vi "Get Available IP List.vi"(7 "ip list property name":string, 8 "error in (no error)":errorcluster, 11 "Item Ref in":T1 format="%.0x") -> (0 "error out":errorcluster, 2 "ips available":string[](array[string]), 3 "Item Ref out":T1 format="%.0x")   [LabVIEW 2017, in "Engine Simulation Toolkit System Explorer.lvlib"]
uses:
  Engine Simulation Toolkit System Explorer.lvlib
  <vilib>/NI Veristand/Custom Device API/Custom Device Item Ref.ctl
  <vilib>/NI Veristand/Custom Device Tools/Custom Device Utility Library/Search Direction.ctl
  Shared/Constants and GUIDs.vi
  <vilib>/NI Veristand/Custom Device Tools/Custom Device Utility Library/NI VeriStand - Search for Item by GUID.vi
  <vilib>/NI Veristand/Custom Device API/Get Item Property (String Array).vi
  <vilib>/NI Veristand/Custom Device Tools/Custom Device Utility Library/Custom Device Utility Library.lvlib
  Shared/Engine Simulation Toolkit Shared.lvlib
  <vilib>/NI Veristand/Custom Device API/Custom Device API.lvlib
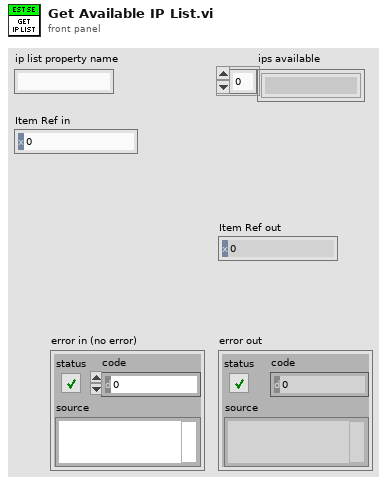
[diagram p1: front panel]
types:
  T1 = typedef "Custom Device API.lvlib/Custom Device Item Ref.ctl" = u64
  T2 = typedef "Custom Device Utility Library.lvlib/Search Direction.ctl" = enum16{"Down", "Up"}
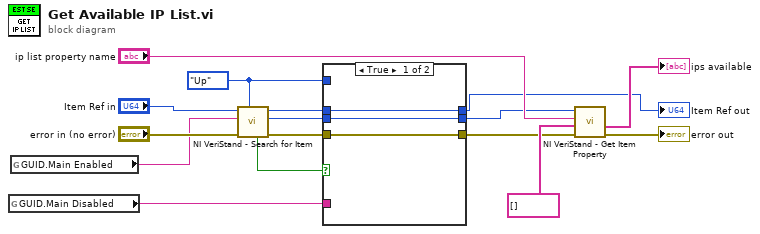
[diagram p0: block diagram]
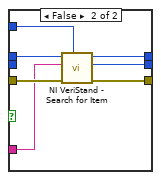
[diagram p2: hidden frame]
diagram:
  w4 = Search_Direction."Up" ("Direction (Down)")
  n1 = global read "Constants and GUIDs.vi" "GUID.Main Disabled"() -> (w5:string)
  n2 = global read "Constants and GUIDs.vi" "GUID.Main Enabled"() -> (w14:string)
  n3 = call-poly <vilib>:"NI VeriStand - Search for Item.vi"("Direction (Down)"=w4, "error in"="error in (no error)", "Item GUID"=w14, "Section Ref in"="Item Ref in") -> ("error out"=w8:errorcluster, "Item Ref"=w6:T1, "Section Ref out"=w7:T1, "Found"=w9:bool)  [unwired: 4 in]
  n4 = case shown="True" w9 {
    tunnel: w8 -> [w19 w26]
    tunnel: w7 -> [w17 w25]
    tunnel: w6 -> [w18 _]
    tunnel: w5 -> [_ w24]
    tunnel: w4 -> [_ w23]
    tunnel: [w18 w22] -> w3
    tunnel: [w17 w21] -> w2
    tunnel: [w19 w20] -> w1
    frame True {
    }
    frame False {
      n5 = call-poly <vilib>:"NI VeriStand - Search for Item.vi"("Direction (Down)"=w23, "error in"=w26, "Item GUID"=w24, "Section Ref in"=w25) -> ("error out"=w20:errorcluster, "Item Ref"=w22:T1, "Section Ref out"=w21:T1)  [unwired: 4 in, 1 out]
    }
  }
  "Item Ref out" <- w2
  n6 = call-poly <vilib>:"NI VeriStand - Get Item Property.vi"("error in (no error)"=w1, "Default Value"=string[] [], "Property Name"="ip list property name", "Item Ref in"=w3) -> ("error out"=→"error out":errorcluster, "Value"=→"ips available":string[])  [unwired: 4 in, 2 out]
